vi "Filter (SubVI).vi"(9 "SamplingInterval":sgl, 10 "IIR filter":T1, 11 "UNDT_Cluster_Data":dbl[](array[numeric])) -> (3 "Filtered X":dbl[](array[numeric]))   [LabVIEW 2017]
uses:
  <vilib>/Analysis/3filter.llb/Butterworth Filter (DBL).vi
  <vilib>/Analysis/3filter.llb/Chebyshev Filter (DBL).vi
  <vilib>/Analysis/3filter.llb/Inverse Chebyshev Filter (DBL).vi
  <vilib>/Analysis/3filter.llb/Elliptic Filter (DBL).vi
  <vilib>/Analysis/3filter.llb/Bessel Filter (DBL).vi
  <vilib>/Analysis/NI_AALBase.lvlib
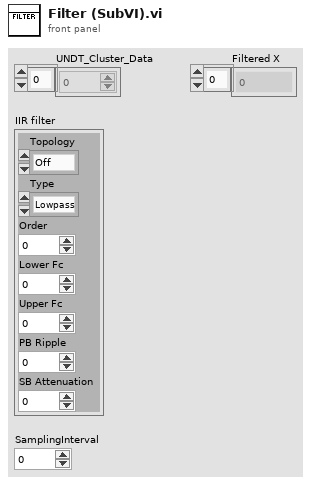
[diagram p1: front panel]
types:
  T1 = cluster{"Topology":enum16{"Off", "Butterworth", "Chebyshev", "Inverse Chebyshev", "Elliptic", "Bessel"}, "Type":enum16{"Lowpass", "Highpass", "Bandpass", "Bandstop"}, "Order":i32, "Lower Fc":dbl, "Upper Fc":dbl, "PB Ripple":dbl, "SB Attenuation":dbl}
  T2 = enum16{"Off", "Butterworth", "Chebyshev", "Inverse Chebyshev", "Elliptic", "Bessel"}
  T3 = enum16{"Lowpass", "Highpass", "Bandpass", "Bandstop"}
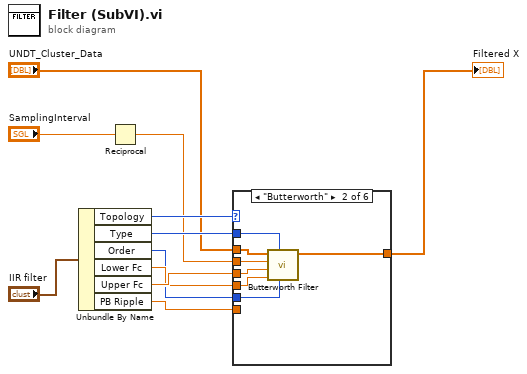
[diagram p0: block diagram]
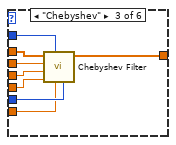
[diagram p3: hidden frame]
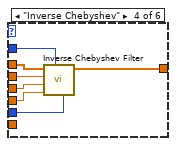
[diagram p4: hidden frame]
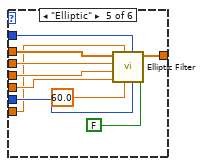
[diagram p5: hidden frame]
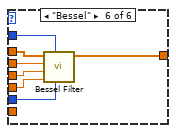
[diagram p6: hidden frame]
diagram:
  n1 = Unbundle By Name("IIR filter") -> ("Topology"=w9:T2, "Type"=w11:T3, "Order"=w2:i32, "Lower Fc"=w3:dbl, "Upper Fc"=w4:dbl, "PB Ripple"=w10:dbl)
  n2 = Reciprocal(x="SamplingInterval") -> (1/x=w1:sgl)
  n3 = case shown="\"Butterworth\"" w9 {
    tunnel: w1 -> [_ w19 w22 w32 w38 w49]
    tunnel: w2 -> [_ w18 w25 w29 w42 w46]
    tunnel: w3 -> [_ w17 w24 w30 w40 w47]
    tunnel: w4 -> [_ w16 w23 w31 w39 w48]
    tunnel: "UNDT_Cluster_Data" -> [w12 w15 w27 w34 w44 w51]
    tunnel: [w12 w14 w26 w33 w43 w45] -> w8
    tunnel: w10 -> [_ _ w21 _ w36 _]
    tunnel: w11 -> [_ w13 w20 w28 w35 w50]
    frame "Off", Default {
    }
    frame "Butterworth" {
      n4 = call-poly <vilib>:"Butterworth Filter.vi"("order"=w18, "filter type"=w13, "low cutoff freq: fl"=w17, "high cutoff freq: fh"=w16, "sampling freq: fs"=w19, "X"=w15) -> ("Filtered X"=w14:dbl[])  [unwired: 2 in, 1 out]
    }
    frame "Chebyshev" {
      n5 = call-poly <vilib>:"Chebyshev Filter.vi"("order"=w25, "ripple(dB)"=w21, "filter type"=w20, "low cutoff freq: fl"=w24, "high cutoff freq: fh"=w23, "sampling freq: fs"=w22, "X"=w27) -> ("Filtered X"=w26:dbl[])  [unwired: 3 in, 1 out]
    }
    frame "Inverse Chebyshev" {
      n6 = call-poly <vilib>:"Inverse Chebyshev Filter.vi"("order"=w29, "filter type"=w28, "low cutoff freq: fl"=w30, "high cutoff freq: fh"=w31, "sampling freq: fs"=w32, "X"=w34) -> ("Filtered X"=w33:dbl[])  [unwired: 4 in, 1 out]
    }
    frame "Elliptic" {
      n7 = call-poly <vilib>:"Elliptic Filter.vi"("init/cont (init:F)"=FALSE, "order"=w42, "filter type"=w35, "stopband attenuation (dB)"=60.0, "passband ripple (dB)"=w36, "low cutoff freq: fl"=w40, "high cutoff freq: fh"=w39, "sampling freq: fs"=w38, "X"=w44) -> ("Filtered X"=w43:dbl[])  [unwired: 1 in, 1 out]
    }
    frame "Bessel" {
      n8 = call-poly <vilib>:"Bessel Filter.vi"("order"=w46, "filter type"=w50, "low cutoff freq: fl"=w47, "high cutoff freq: fh"=w48, "sampling freq: fs"=w49, "X"=w51) -> ("Filtered X"=w45:dbl[])  [unwired: 2 in, 1 out]
    }
  }
  "Filtered X" <- w8
